vi "Cluster to String Array.vi"(1 "Account Information":T1) -> (0 "Array":string[](array[string]))   [LabVIEW 2020, in "IInfoable.lvclass"]
uses:
  IInfoable.lvclass
  Account Information STYP.ctl
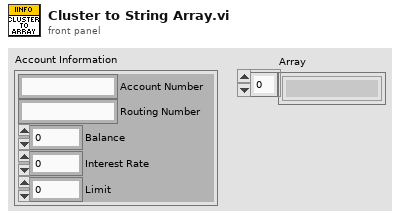
[diagram p1: front panel]
types:
  T1 = typedef "IInfoable.lvclass/Account Information STYP.ctl" = cluster{"Account Number":string, "Routing Number":string, "Balance":dbl, "Interest Rate":dbl, "Limit":dbl}
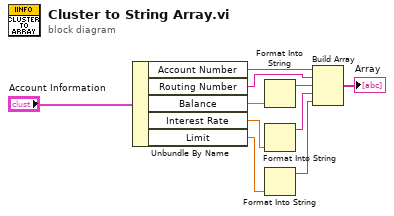
[diagram p0: block diagram]
diagram:
  n1 = Unbundle By Name("Account Information") -> ("Account Number"=w6:string, "Routing Number"=w5:string, "Balance"=w9:dbl, "Interest Rate"=w8:dbl, "Limit"=w7:dbl)
  n2 = Format Into String(w9) -> (resulting string=w4:string)  [unwired: 3 in, 1 out]
  n3 = Format Into String(w8) -> (resulting string=w3:string)  [unwired: 3 in, 1 out]
  n4 = Format Into String(w7) -> (resulting string=w2:string)  [unwired: 3 in, 1 out]
  n5 = Build Array(w6, w5, w4, w3, w2) -> (→"Array":string[])
